vi "Configure TV Trig Custom.vi"(8 "error in (no error)":errorcluster {"code" format="%.0x"}, 9 "Custom Scan Rate (15 - 20 KHz)":i32(slide), 10 "Custom Format (Interlaced)":i32(slide), 11 "VISA Resource Name":refnum<visa-resource-name>) -> (0 "error out":errorcluster {"code" format="%.0x"}, 3 "VISA Resource Name Out":refnum<visa-resource-name>)   [LabVIEW 2010, in "Tektronix TDS 3000 Series.lvlib"]
doc: "This VI configures the custom triggering mode.\n\nNotes:\n\n(1) This VI is effective only if TV Trigger Signal Format in Configure TV Trigger Source is selected as Custom"
uses:
  <instrlib>/Tektronix TDS 3000 Series/Tektronix TDS 3000 Series.lvlib
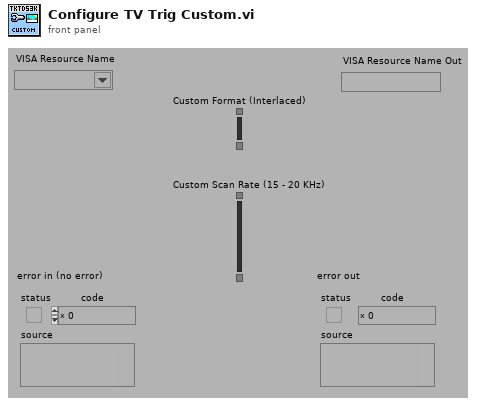
[diagram p1: front panel]
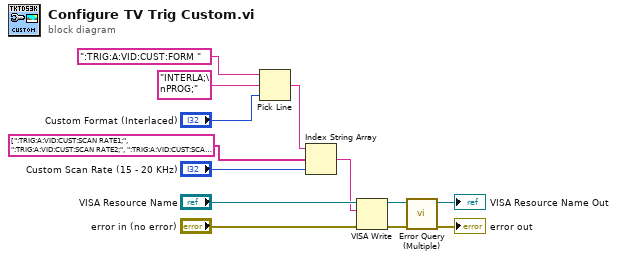
[diagram p0: block diagram]
diagram:
  n1 = Pick Line(string ("")=":TRIG:A:VID:CUST:FORM " ("format string"), multi-line string="INTERLA;\nPROG;", line index="Custom Format (Interlaced)") -> (output string=w8:string)
  n2 = Index String Array(1:"Custom Scan Rate (15 - 20 KHz)", 2:string[] [":TRIG:A:VID:CUST:SCAN RATE1;", ":TRIG:A:VID:CUST:SCAN RATE2;", ":TRIG:A:VID:CUST:SCAN RATE3;", ":TRIG:A:VID:CUST:SCAN RATE4;", ":TRIG:A:VID:CUST:SCAN RATE5;"] ("string array"), 3:w8) -> (0:w5:string)
  n3 = VISA Write(VISA resource name="VISA Resource Name", write buffer=w5, error in (no error)="error in (no error)") -> (VISA resource name out=w4:refnum<visa-resource-name>, error out=w3:errorcluster)  [unwired: 1 out]
  n4 = call <instrlib>:"Error Query (Multiple).vi"("error in (no error)"=w3, "VISA Resource Name"=w4) -> ("error out"=→"error out":errorcluster, "VISA Resource Name Out"=→"VISA Resource Name Out":refnum<visa-resource-name>)  [unwired: 6 in, 2 out]
